vi "FGV Gasteiler.vi"(0 "Gasteiler Daten":T5={"Gasteiler"="", "Gasteiler Stufen"=128, "Gasteiler Type"=0, "Konfig Gasteiler"=0, "Gasteiler Span Eingänge"=128} {"Gasteiler Span Eingänge" items=["0", "1", "2", "3", "4", "5", "6", "7", "8", "9", "10"]; "Konfig Gasteiler" items=["----"=10000]; "Gasteiler Type" items=["LNI", "Analog-Display", "AVL GDU", "Horiba GDC", "HovaCal", "Horiba SGD 710C"]; "Gasteiler Stufen" items=["10"=10, "11"=11, "16"=16, "32"=32, "64"=64, "128"=128, "256"=256, "500"=500, "1000"=1000]}, 1 "TCP":T1, 3 "Anforderung":bool, 4 "Serielle Parameter":T3={"VISA resource name"="COM1", "baud rate"=38400, "data bits"=8, "parity"=0, "stop bits"=10, "flow control"=0} {"flow control" items=["None"=0, "XON/XOFF"=1, "RTS/CTS"=2, "DTR/DSR"=4]; "stop bits" items=["1.0"=10, "1.5"=15, "2.0"=20]; "parity" items=["None", "Odd", "Even", "Mark", "Space"]; "data bits" min=5 max=8 step=1}, 5 "error in (no error)":errorcluster caption="Fehler (Eingang, kein Fehler)", 6 "MB-Endwert":u32, 7 "Aufzeichnung Start":bool, 11 "Aktionen":T4) -> (12 "MB-Endwert":u32, 13 "Aufzeichnung Start":bool, 14 "Gasteiler Daten":T5={"Gasteiler"="", "Gasteiler Stufen"=128, "Gasteiler Type"=0, "Konfig Gasteiler"=0, "Gasteiler Span Eingänge"=128} {"Gasteiler Span Eingänge" items=["0", "1", "2", "3", "4", "5", "6", "7", "8", "9", "10"]; "Konfig Gasteiler" items=["----"=10000]; "Gasteiler Type" items=["LNI", "Analog-Display", "AVL GDU", "Horiba GDC", "HovaCal", "Horiba SGD 710C"]; "Gasteiler Stufen" items=["10"=10, "11"=11, "16"=16, "32"=32, "64"=64, "128"=128, "256"=256, "500"=500, "1000"=1000]}, 15 "TCP":T1, 16 "Gasteiler Type":T2 items=["LNI", "Analog-Display", "AVL GDU", "Horiba GDC", "HovaCal", "Horiba SGD 710C"], 17 "Anforderung":bool, 18 "Serielle Parameter":T3={"VISA resource name"="COM1", "baud rate"=38400, "data bits"=8, "parity"=0, "stop bits"=10, "flow control"=0} {"flow control" items=["None"=0, "XON/XOFF"=1, "RTS/CTS"=2, "DTR/DSR"=4]; "stop bits" items=["1.0"=10, "1.5"=15, "2.0"=20]; "parity" items=["None", "Odd", "Even", "Mark", "Space"]; "data bits" min=5 max=8 step=1}, 19 "error out":errorcluster caption="Fehler (Ausgang)")   [LabVIEW 2020, in "Linearisierung v2.lvlib" / "Gasteiler.lvlib"]
uses:
  Gasteiler.lvlib
  Gasteiler Daten.ctl
  Visualisierungs Elemente/String - Eingabefeld.ctl
  Gasteiler Stufen.ctl
  GasteilerType.ctl
  Seiten/System Einstellungen V2/Gasteiler Auswahl.ctl
  Aktionen FGV Gasteiler Daten.ctl
  AK-Schnittstelle/Serielle Parameter.ctl
  Allgemein/allgemeine Sub-VIs.lvlib
  AK-Schnittstelle/AK Seriell/AK Seriell.lvlib
  Linearisierung v2.lvlib
  Seiten/System Einstellungen V2/System Einstellungen V2.lvlib
panel:
  # "SPAN Eingänge:"
  # "SPAN Eingänge:"
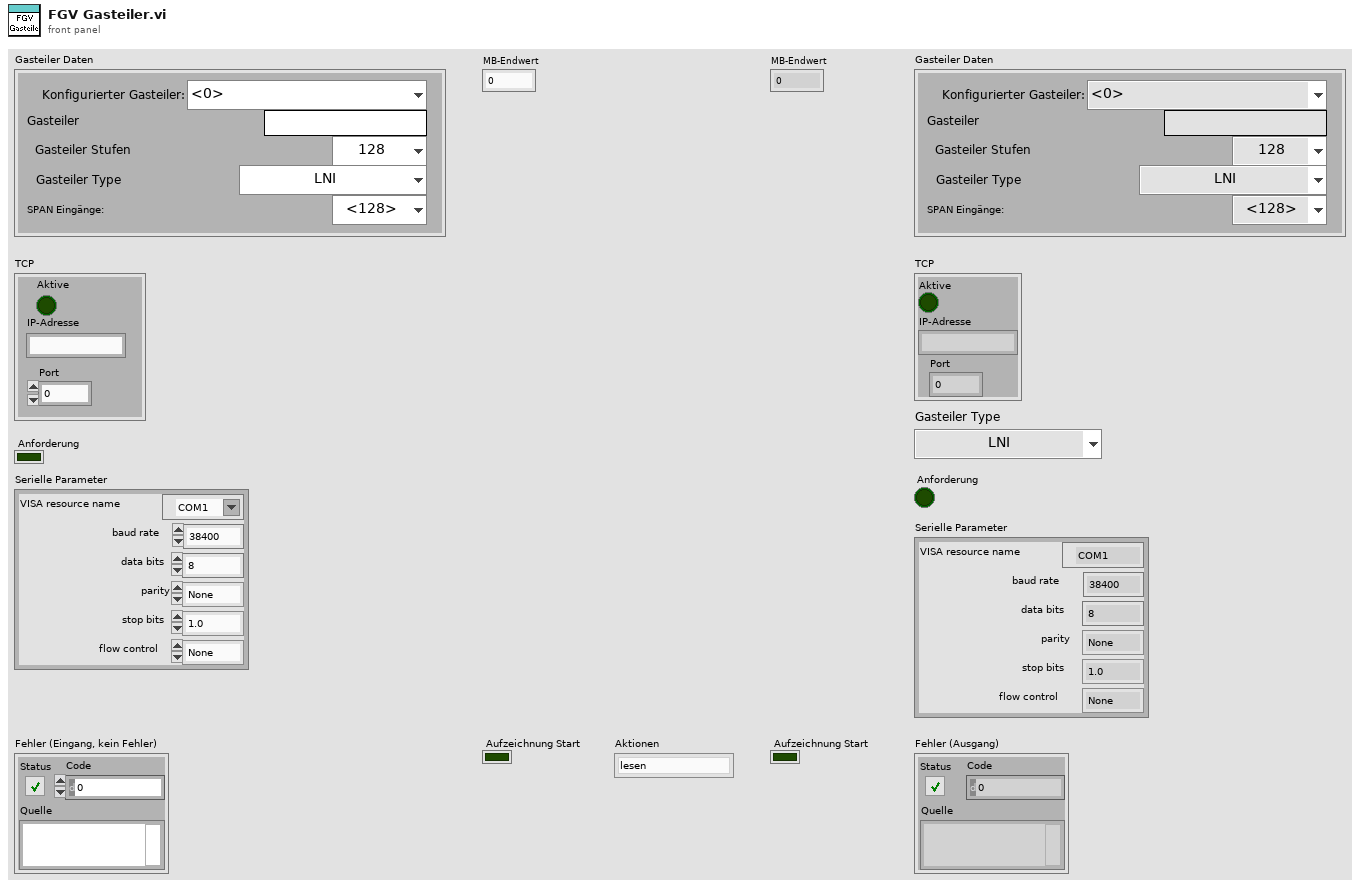
[diagram p1: front panel]
types:
  T1 = cluster{"Aktive":bool, "IP-Adresse":string, "Port":u16}
  T2 = typedef "Linearisierung v2.lvlib/GasteilerType.ctl" = u16
  T3 = typedef "AK-Schnittstelle.lvlib/AK Seriell.lvlib/Serielle Parameter.ctl" = cluster{"VISA resource name":refnum<visa-resource-name>, "baud rate":u32, "data bits":u16, "parity":u16, "stop bits":u16, "flow control":u16}
  T4 = typedef "Linearisierung v2.lvlib/Gasteiler.lvlib/Aktionen FGV Gasteiler Daten.ctl" = enum16{"lesen", "Gasteiler Daten", "Seriellen Param.", "MB-Endwert", "laden", "speichern", "Anforderung", "TCP", "Aufzeichnung Start"}
  T5 = typedef "Linearisierung v2.lvlib/Gasteiler.lvlib/Gasteiler Daten.ctl" = cluster{"Gasteiler":T6, "Gasteiler Stufen":T7, "Gasteiler Type":T2, "Konfig Gasteiler":T8, "Gasteiler Span Eingänge":u16}
  T6 = typedef "String - Eingabefeld.ctl" = string
  T7 = typedef "Linearisierung v2.lvlib/Gasteiler.lvlib/Gasteiler Stufen.ctl" = u16
  T8 = typedef "System Einstellungen V2.lvlib/Gasteiler Auswahl.ctl" = u16
  T9 = cluster{"Gasteiler Daten":T5, "Serielle Parameter":T3, "TCP":cluster{"Aktive":bool, "IP-Adresse":string, "Port":u16}}
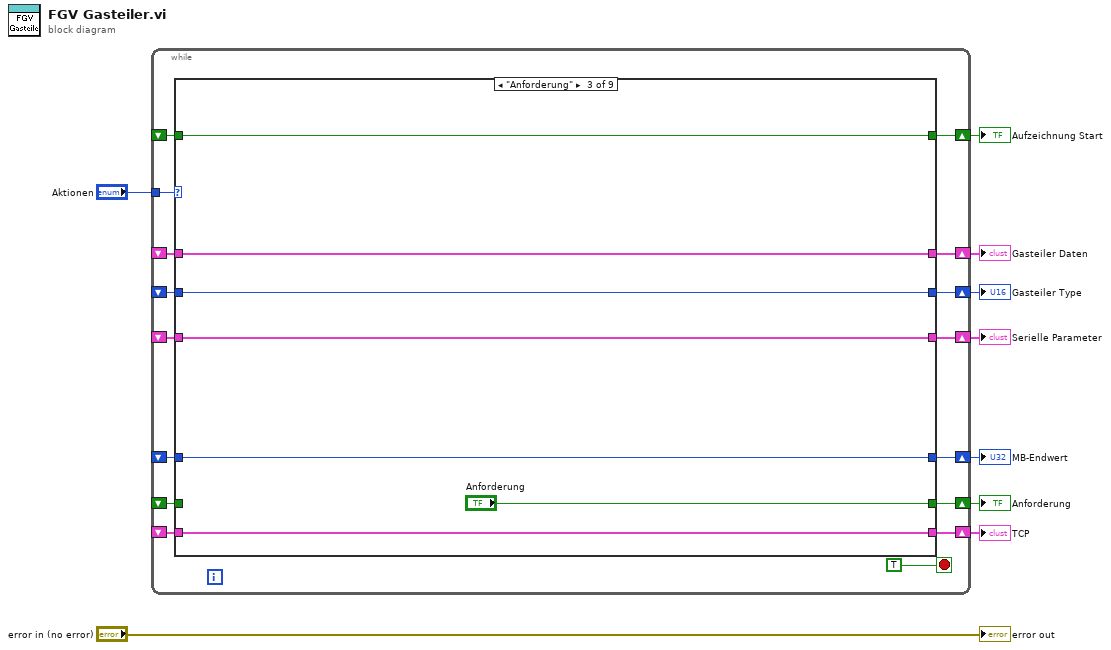
[diagram p0: block diagram]
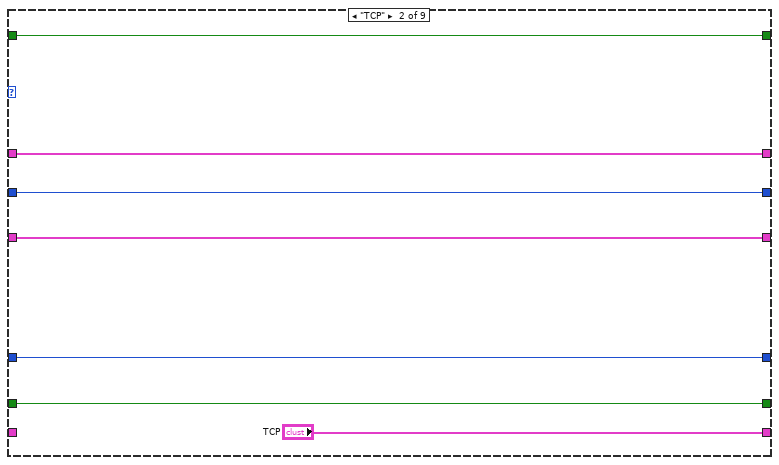
[diagram p3: hidden frame]
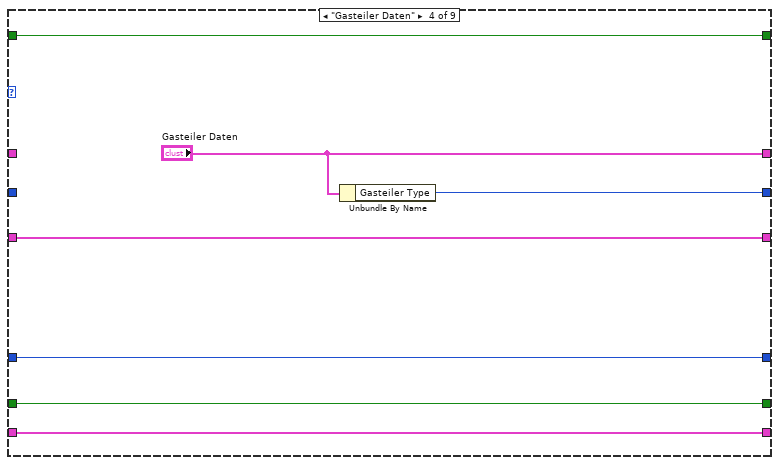
[diagram p4: hidden frame]
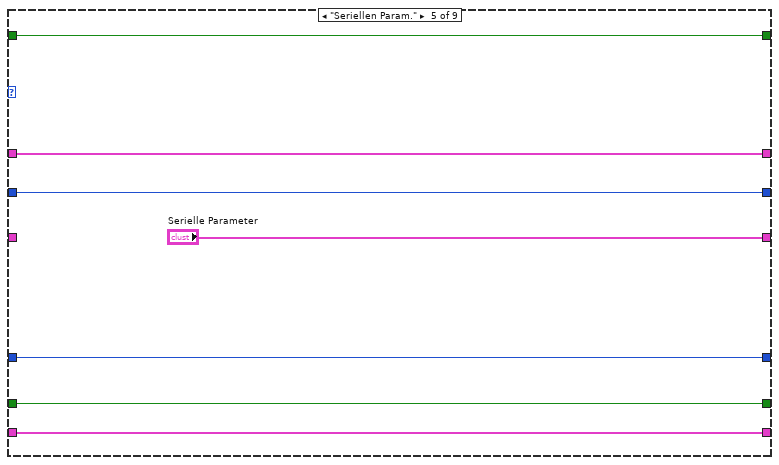
[diagram p5: hidden frame]
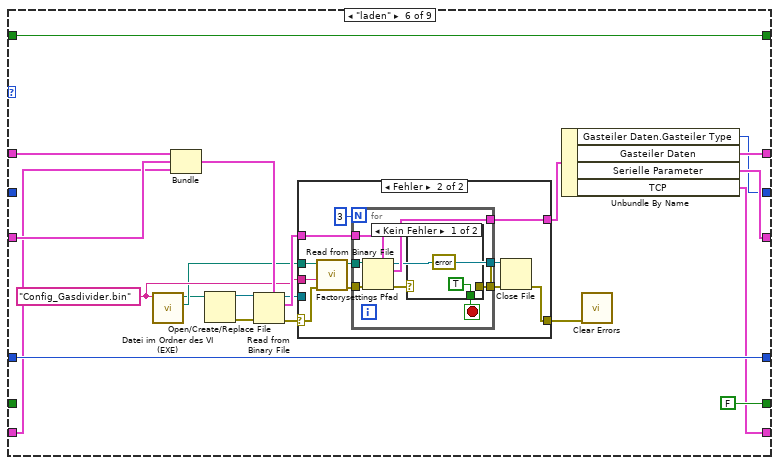
[diagram p6: hidden frame]
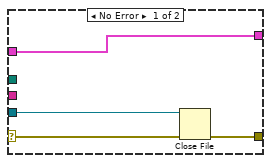
[diagram p7: hidden frame]
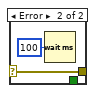
[diagram p8: hidden frame]
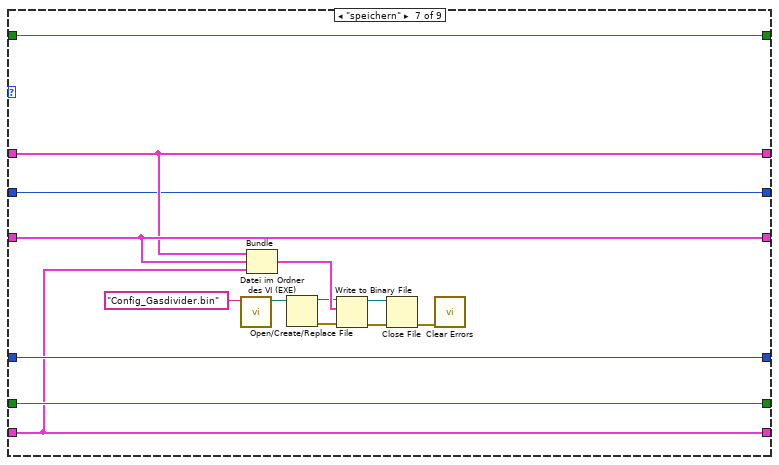
[diagram p9: hidden frame]
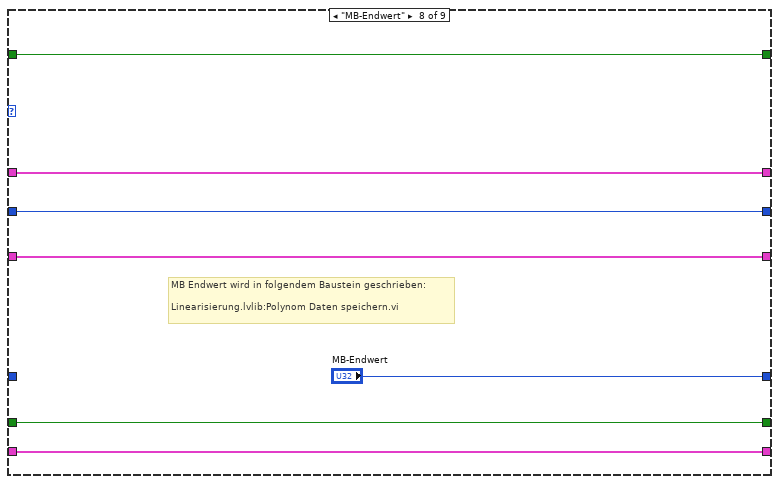
[diagram p10: hidden frame]
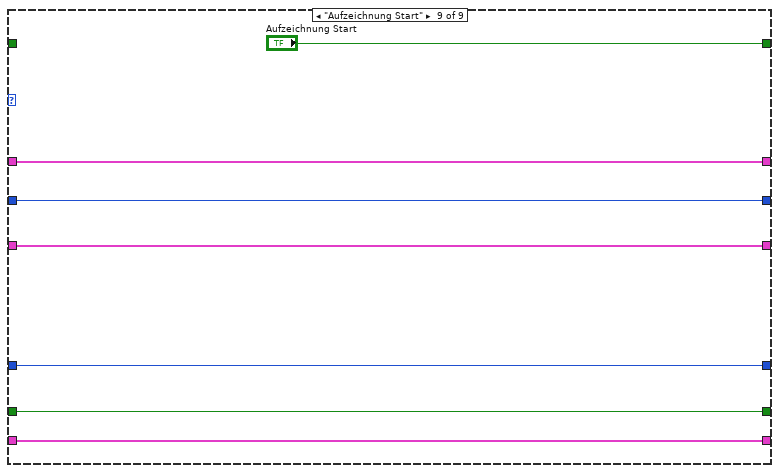
[diagram p11: hidden frame]
diagram:
  n1 = while {
    shift-right: [w22] -> w8
    shift-left: _ -> [w23]
    tunnel: "Aktionen" -> [w24]
    shift-right: [w20] -> w7
    shift-left: _ -> [w21]
    shift-right: [w19] -> w6
    shift-left: _ -> [w18]
    shift-right: [w17] -> w5
    shift-left: _ -> [w16]
    shift-right: [w15] -> w4
    shift-left: _ -> [w14]
    shift-right: [w13] -> w3
    shift-left: _ -> [w12]
    shift-right: [w11] -> w2
    shift-left: _ -> [w10]
    stop <- TRUE stop-if-true
    n2 = case shown="\"Anforderung\"" w24 {
      tunnel: w23 -> [w32 w39 w46 _ w59 w80 w121 w128 w136]
      tunnel: [w32 w39 w46 "Gasteiler Daten" w59 w76 w121 w128 w136] -> w22
      tunnel: w21 -> [w31 w38 w45 w53 _ w79 w122 w129 w134]
      tunnel: [w31 w38 w45 w53 "Serielle Parameter" w78 w122 w129 w134] -> w20
      tunnel: [w30 w37 w44 w52 w58 w77 w119 "MB-Endwert" w133] -> w19
      tunnel: w18 -> [w30 w37 w44 w52 w58 w77 w119 _ w133]
      tunnel: [w29 w36 w43 w50 w57 w75 w118 w127 w135] -> w17
      tunnel: w16 -> [w29 w36 w43 _ w57 _ w118 w127 w135]
      tunnel: [w28 w35 "Anforderung" w49 w56 FALSE ("Anforderung") w117 w126 w132] -> w15
      tunnel: w14 -> [w28 w35 _ w49 w56 _ w117 w126 w132]
      tunnel: [w27 "TCP" w41 w48 w55 w72 w116 w125 w131] -> w13
      tunnel: w12 -> [w27 _ w41 w48 w55 w73 w116 w125 w131]
      tunnel: [w26 w33 w40 w47 w54 w71 w115 w124 "Aufzeichnung Start"] -> w11
      tunnel: w10 -> [w26 w33 w40 w47 w54 w71 w115 w124 _]
      frame "lesen", Default {
      }
      frame "TCP" {
      }
      frame "Anforderung" {
      }
      frame "Gasteiler Daten" {
        n3 = Unbundle By Name("Gasteiler Daten") -> ("Gasteiler Type"=w50:T2)
      }
      frame "Seriellen Param." {
      }
      frame "laden" {
        w65 = "Config_Gasdivider.bin" ("Dateiname")
        n4 = call "Datei im Ordner des VI (EXE).vi"("Dateiname"=w65) -> ("Ordner des Haupt-VIs"=w64:path, "Dateipfad im Ordner des Haupt-VIs"=w62:path)  [unwired: 8 in, 1 out]
        n5 = Bundle("Gasteiler Daten"=w80, "Serielle Parameter"=w79, "TCP"=w73) -> (w81:T9)  [unwired: 1 in]
        n6 = Open/Create/Replace File(file path (use dialog)=w62) -> (refnum out=w61:refnum<file>, error out=w63:errorcluster)  [unwired: 5 in, 1 out]
        n7 = Read from Binary File(5:w81, 8:w63, 11:w61) -> (0:w67:errorcluster, 2:w69:T9, 3:w68:refnum<file>)  [unwired: 4 out]
        n8 = case shown="Fehler" w67 {
          selector: w67 -> [w84 w88]
          tunnel: w64 -> [_ w89]
          tunnel: w69 -> [w85 w87]
          tunnel: [w85 w95] -> w70
          tunnel: [w82 w93] -> w66
          tunnel: w68 -> [w83 _]
          tunnel: w65 -> [_ w86]
          frame No Error {
            n9 = Close File(refnum=w83, error in=w84) -> (error out=w82:errorcluster)  [unwired: 1 out]
          }
          frame Error {
            n10 = call "Factorysettings Pfad.vi"("error in (no error)"=w88, "Dateiname"=w86, "Ordner des Haupt-VIs"=w89) -> ("error out"=w90:errorcluster, "Pfad Factorysettings"=w91:path)  [unwired: 7 in]
            n11 = for {
              N: 3 -> [_]
              tunnel: w90 -> [w102]
              tunnel: w91 -> [w101]
              tunnel: [w100] -> w95
              tunnel: [w99] -> w94
              tunnel: [w98] -> w92
              tunnel: w87 -> [w97]
              stop <- w103 stop-if-true
              n12 = Read from Binary File(5:w97, 8:w102, 11:w101) -> (0:w104:errorcluster, 2:w100:T9, 3:w98:refnum<file>)  [unwired: 3 in, 1 out]
              n13 = case shown="Kein Fehler" w104 {
                selector: w104 -> [_ w107]
                tunnel: [TRUE _] -> w103
                tunnel: [errorcluster {"status"=FALSE, "code"=0, "source"=""} ("error IO") w107] -> w99
                frame No Error {
                }
                frame Error {
                  n14 = Wait (ms)(milliseconds to wait=u32 100 ("Zu wartende ms")) -> ()  [unwired: 1 out]
                }
              }
            }
            n15 = Close File(refnum=w92, error in=w94) -> (error out=w93:errorcluster)  [unwired: 1 out]
          }
        }
        n16 = Unbundle By Name(w70) -> ("Gasteiler Daten.Gasteiler Type"=w75:T2, "Gasteiler Daten"=w76:T5, "Serielle Parameter"=w78:T3, "TCP"=w72:T1)
        n17 = call <vilib>:"Clear Errors.vi"("error in (no error)"=w66) -> ()  [unwired: 5 in, 2 out]
      }
      frame "speichern" {
        n18 = call "Datei im Ordner des VI (EXE).vi"("Dateiname"="Config_Gasdivider.bin") -> ("Dateipfad im Ordner des Haupt-VIs"=w113:path)  [unwired: 8 in, 2 out]
        n19 = Bundle("Gasteiler Daten"=w121, "Serielle Parameter"=w122, "TCP"=w116) -> (w120:T9)  [unwired: 1 in]
        n20 = Open/Create/Replace File(file path (use dialog)=w113) -> (refnum out=w112:refnum<file>, error out=w114:errorcluster)  [unwired: 5 in, 1 out]
        n21 = Write to Binary File(file (use dialog)=w112, data=w120, error in=w114) -> (refnum out=w110:refnum<file>, error out=w111:errorcluster)  [unwired: 1 in, 3 out]
        n22 = Close File(refnum=w110, error in=w111) -> (error out=w109:errorcluster)  [unwired: 1 out]
        n23 = call <vilib>:"Clear Errors.vi"("error in (no error)"=w109) -> ()  [unwired: 5 in, 2 out]
      }
      frame "MB-Endwert" {
        # "MB Endwert wird in folgendem Baustein geschrieben:\n\nLinearisierung.lvlib:Polynom Daten speichern.vi"
      }
      frame "Aufzeichnung Start" {
      }
    }
  }
  "Gasteiler Daten" <- w8
  "Serielle Parameter" <- w7
  "MB-Endwert" <- w6
  "Gasteiler Type" <- w5
  "Anforderung" <- w4
  "TCP" <- w3
  "Aufzeichnung Start" <- w2
  "error out" <- "error in (no error)"
